vi "Practica 10.vi"() -> ()   [LabVIEW 2018]
uses:
  <vilib>/LabVIEW Interface for Arduino/Type Defs/Pin Mode.ctl
  <vilib>/LabVIEW Interface for Arduino/Type Defs/Connection Type.ctl
  <vilib>/LabVIEW Interface for Arduino/Type Defs/Board Type.ctl
  <vilib>/LabVIEW Interface for Arduino/LabVIEW Interface for Arduino.lvlib
panel:
  in  "VERDE":dbl
  in  "AMARILLO":dbl
  in  "ROJO":dbl
  out "Rojo":bool
  out "Amarillo":bool
  out "Verde":bool
  in  "Detener":bool
  # "Practica 10: Semaforo Ajustable"
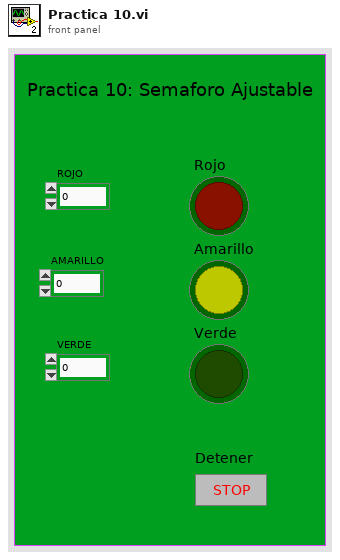
[diagram p1: front panel]
types:
  T1 = typedef "LabVIEW Interface for Arduino.lvlib/Board Type.ctl" = enum16{"Uno", "Dimuelanove w/Atmega 328", "Mega 2560"}
  T2 = typedef "LabVIEW Interface for Arduino.lvlib/Connection Type.ctl" = enum8{"USB / Serial", "XBEE", "BlueSmirf (Bluetooth)"}
  T3 = typedef "LabVIEW Interface for Arduino.lvlib/Pin Mode.ctl" = enum8{"Input", "Output"}
  T4 = typedef "LabVIEW Interface for Arduino.lvlib/Arduino Resource.ctl" = cluster{"VISA resource":refnum<visa-resource-name>, "Board Type":T1, "Connection Type":enum8{"USB / Serial"}, "Bytes Per Packet (15)":u8}
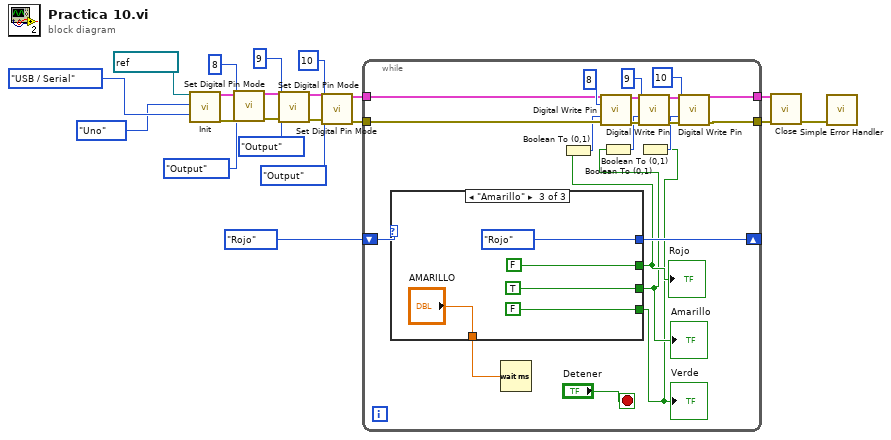
[diagram p0: block diagram]
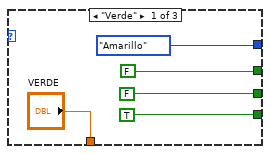
[diagram p2: hidden frame]
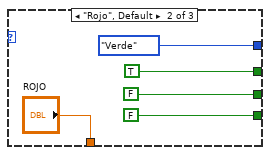
[diagram p3: hidden frame]
diagram:
  n1 = call <vilib>:"Init.vi"("VISA resource"=refnum<visa-resource-name> "COM9", "Board Type (Uno)"=Board_Type."Uno", "Connection Type (USB/Serial)"=Connection_Type."USB / Serial") -> ("Arduino Resource"=w21:T4, "error out"=w20:errorcluster)  [unwired: 15 in]
  n2 = call <vilib>:"Set Digital Pin Mode.vi"("Arduino Resource"=w21, "Digital I/O Pin"=u8 8, "Pin Mode (Input)"=Pin_Mode."Output", "error in"=w20) -> ("Arduino Resource"=w19:T4, "error out"=w18:errorcluster)  [unwired: 10 in]
  n3 = call <vilib>:"Set Digital Pin Mode.vi"("Arduino Resource"=w19, "Digital I/O Pin"=u8 9, "Pin Mode (Input)"=Pin_Mode."Output", "error in"=w18) -> ("Arduino Resource"=w17:T4, "error out"=w16:errorcluster)  [unwired: 10 in]
  n4 = call <vilib>:"Set Digital Pin Mode.vi"("Arduino Resource"=w17, "Digital I/O Pin"=u8 10, "Pin Mode (Input)"=Pin_Mode."Output", "error in"=w16) -> ("Arduino Resource"=w8:T4, "error out"=w7:errorcluster)  [unwired: 10 in]
  n5 = while {
    shift-right: [w40] -> _
    shift-left: enum16{"Rojo", "Amarillo", "Verde"}."Rojo" -> [w41]
    tunnel: w8 -> [w31]
    tunnel: w7 -> [w30]
    tunnel: [w23] -> w6
    tunnel: [w22] -> w5
    stop <- "Detener" stop-if-true
    n6 = case shown="\"Amarillo\"" w41 {
      tunnel: [enum16{"Rojo", "Amarillo", "Verde"}."Amarillo" enum16{"Rojo", "Amarillo", "Verde"}."Verde" enum16{"Rojo", "Amarillo", "Verde"}."Rojo"] -> w40
      tunnel: [FALSE TRUE FALSE] -> w26
      tunnel: [FALSE FALSE TRUE] -> w25
      tunnel: [TRUE FALSE FALSE] -> w24
      tunnel: ["VERDE" "ROJO" "AMARILLO"] -> w39
      frame "Verde" {
      }
      frame "Rojo", Default {
      }
      frame "Amarillo" {
      }
    }
    "Rojo" <- w26
    "Amarillo" <- w25
    "Verde" <- w24
    n7 = Wait (ms)(milliseconds to wait=w39) -> ()  [unwired: 1 out]
    n8 = Boolean To (0,1)(Boolean=w26) -> (0, 1=w29:i16)
    n9 = call <vilib>:"Digital Write Pin.vi"("Arduino Resource"=w31, "Digital I/O Pin (0)"=u8 8, "Value (0)"=w29, "error in"=w30) -> ("Arduino Resource"=w38:T4, "error out"=w35:errorcluster)  [unwired: 10 in]
    n10 = Boolean To (0,1)(Boolean=w25) -> (0, 1=w27:i16)
    n11 = call <vilib>:"Digital Write Pin.vi"("Arduino Resource"=w38, "Digital I/O Pin (0)"=u8 9, "Value (0)"=w27, "error in"=w35) -> ("Arduino Resource"=w37:T4, "error out"=w36:errorcluster)  [unwired: 10 in]
    n12 = Boolean To (0,1)(Boolean=w24) -> (0, 1=w28:i16)
    n13 = call <vilib>:"Digital Write Pin.vi"("Arduino Resource"=w37, "Digital I/O Pin (0)"=u8 10, "Value (0)"=w28, "error in"=w36) -> ("Arduino Resource"=w23:T4, "error out"=w22:errorcluster)  [unwired: 10 in]
  }
  n14 = call <vilib>:"Close.vi"("Arduino Resource"=w6, "error in"=w5) -> ("error out"=w4:errorcluster)  [unwired: 13 in]
  n15 = call <vilib>:"Simple Error Handler.vi"("error in (no error)"=w4) -> ()  [unwired: 4 in, 5 out]
